vi "vi_lib_path.vi"() -> (3 "transition.llb":path)   [LabVIEW 2017, in "GetSetShared.lvlib"]
uses:
  <vilib>/express/express signal manip/GetorSetDDTAttributes/Shared VIs/GetSetShared.lvlib
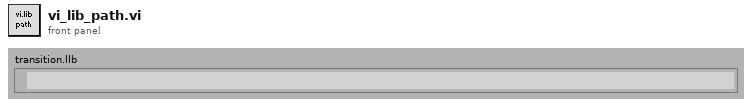
[diagram p1: front panel]
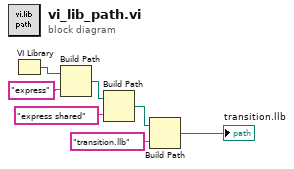
[diagram p0: block diagram]
diagram:
  n1 = VI Library() -> (path=w2:path)
  n2 = Build Path(base path=w2, name or relative path="express") -> (appended path=w3:path)
  n3 = Build Path(base path=w3, name or relative path="express shared") -> (appended path=w1:path)
  n4 = Build Path(base path=w1, name or relative path="transition.llb") -> (appended path=→"transition.llb":path)
